vi "Automatic Error Handling.vi"() -> ()   [LabVIEW 2020]
uses:
  <vilib>/DAQmx/read.llb/DAQmx Read (Analog 1D DBL 1Chan NSamp).vi
  <vilib>/DAQmx/create/channels.llb/DAQmx Create Channel (AI-Acceleration-Accelerometer).vi
  <vilib>/DAQmx/configure/timing.llb/DAQmx Timing (Sample Clock).vi
  <vilib>/DAQmx/miscellaneous.llb/DAQmx Fill In Error Info.vi
panel:
  out "Acceleration Data - Graph":dbl[](graph)
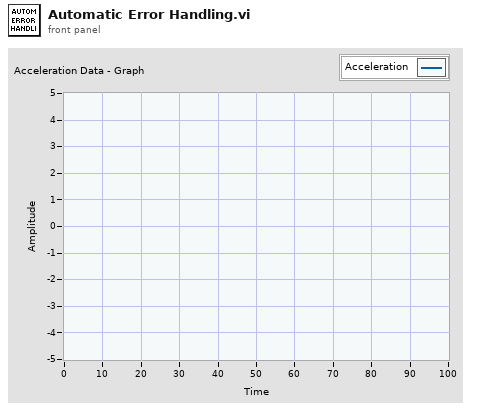
[diagram p1: front panel]
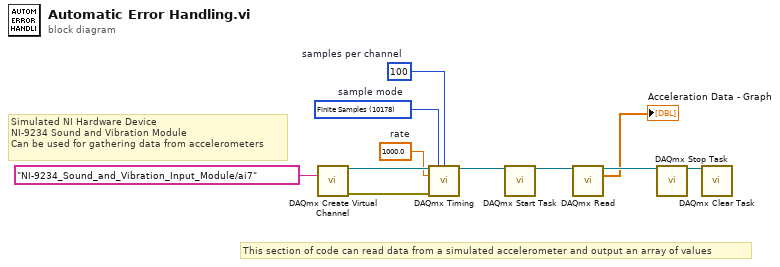
[diagram p0: block diagram]
diagram:
  w3 = 1000.0  # rate
  w4 = 100  # samples per channel
  w5 = 10178 items=["Finite Samples"=10178, "Continuous Samples"=10123, "Hardware Timed Single Point"=12522]  # sample mode
  # "This section of code can read data from a simulated accelerometer and output an array of values"
  # "Simulated NI Hardware Device\nNI-9234 Sound and Vibration Module\nCan be used for gathering data from accelerometers"
  n1 = call-poly <vilib>:"DAQmx Create Virtual Channel.vi"("physical channels"=tag "NI-9234_Sound_and_Vibration_Input_Module/ai7") -> ("task out"=w7:refnum<k21>, "error out"=w1:errorcluster)  [unwired: 13 in]
  n2 = call-poly <vilib>:"DAQmx Timing.vi"("task/channels in"=w7, "sample mode"=w5, "samples per channel"=w4, "rate"=w3, "error in"=w1) -> ("task out"=w6:refnum<k21>)  [unwired: 9 in, 1 out]
  n3 = call <vilib>:"DAQmx Start Task.vi"("task/channels in"=w6) -> ("task out"=w11:refnum<k21>)  [unwired: 13 in, 1 out]
  n4 = call-poly <vilib>:"DAQmx Read.vi"("task/channels in"=w11) -> ("task out"=w9:refnum<k21>, "data"=→"Acceleration Data - Graph":dbl[])  [unwired: 12 in, 1 out]
  n5 = call <vilib>:"DAQmx Stop Task.vi"("task/channels in"=w9) -> ("task out"=w10:refnum<k21>)  [unwired: 13 in, 1 out]
  n6 = call <vilib>:"DAQmx Clear Task.vi"("task in"=w10) -> ()  [unwired: 14 in, 1 out]
